vi "Exercício 4.vi"() -> ()   [LabVIEW 2016]
uses:
  bcf247fc-8029-4b24-a8d5-3c8da93c177a.vi
  <vilib>/numeric/Random Number (Range) DBL.vi
  <vilib>/picture/cartesn2.llb/XY Plot Type.ctl
panel:
  in  "dimensions (w,h)":cluster{"width":i16, "height":i16}={"width"=500, "height"=350}
  in  "cartesian grid cosmetics":T1={"line color"=12369084, "text color"=0, "tick length(3)"=3, "crossing axes"=FALSE, "visible grid?"=TRUE}
  in  "cartesian axis attributes":T2={"x minimum"=0.0, "x maximum"=0.0, "x log?"=FALSE, "x precision"=1, "x format"=enum."Scientific", "y minimum"=0.0, "y maximum"=0.0, "y log?"=FALSE, "y precision"=1, "y format"=enum."Decimal"} {"x minimum" format="%0.2f"; "x maximum" format="%0.2f"; "y minimum" format="%0.2f"; "y maximum" format="%0.2f"}
  in  "Slide":dbl(slide) scale=0.0..300.0
  out "Número Aleatório":dbl
  in  "XY plot cosmetics":T4={"plot color"=0, "XY plot type"=enum."connected circles", "baseline"=0.0} {"baseline" format="%0.2f"}
  out "Temperatura vs Tempo":picture
  in  "stop":bool
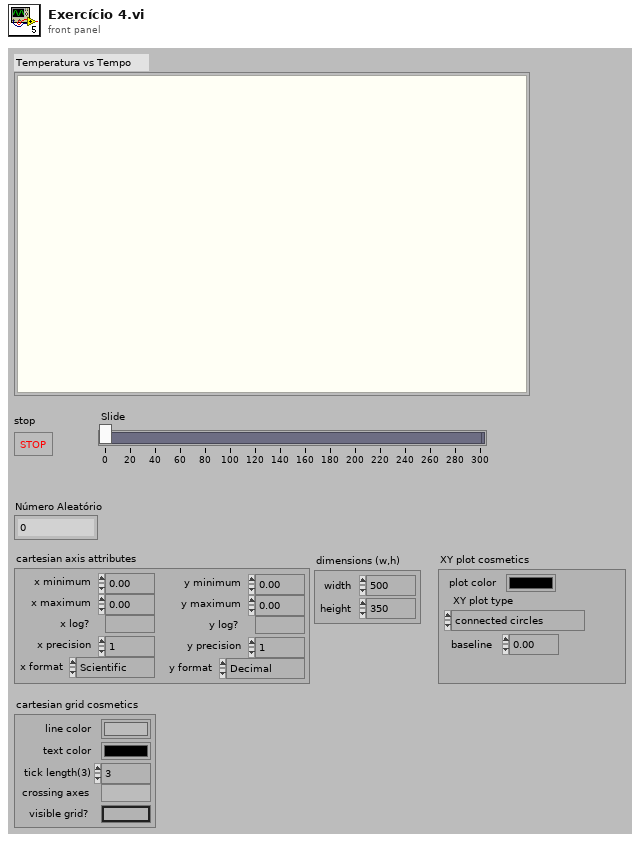
[diagram p1: front panel]
types:
  T1 = cluster{"line color":u32, "text color":u32, "tick length(3)":i16, "crossing axes":bool, "visible grid?":bool}
  T2 = cluster{"x minimum":dbl, "x maximum":dbl, "x log?":bool, "x precision":u8, "x format":enum8{"Decimal", "Scientific", "Engineering", "Binary", "Octal", "Hex"}, "y minimum":dbl, "y maximum":dbl, "y log?":bool, "y precision":u8, "y format":enum8{"Decimal", "Scientific", "Engineering", "Binary", "Octal", "Hex"}}
  T3 = typedef "XY Plot Type.ctl" = enum16{"points", "squares", "circles", "connected points", "connected squares", "connected circles", "comb plot", "sized scatter plot", "sized-colored scatter plot", "min-max lines"}
  T4 = cluster{"plot color":u32, "XY plot type":T3, "baseline":dbl}
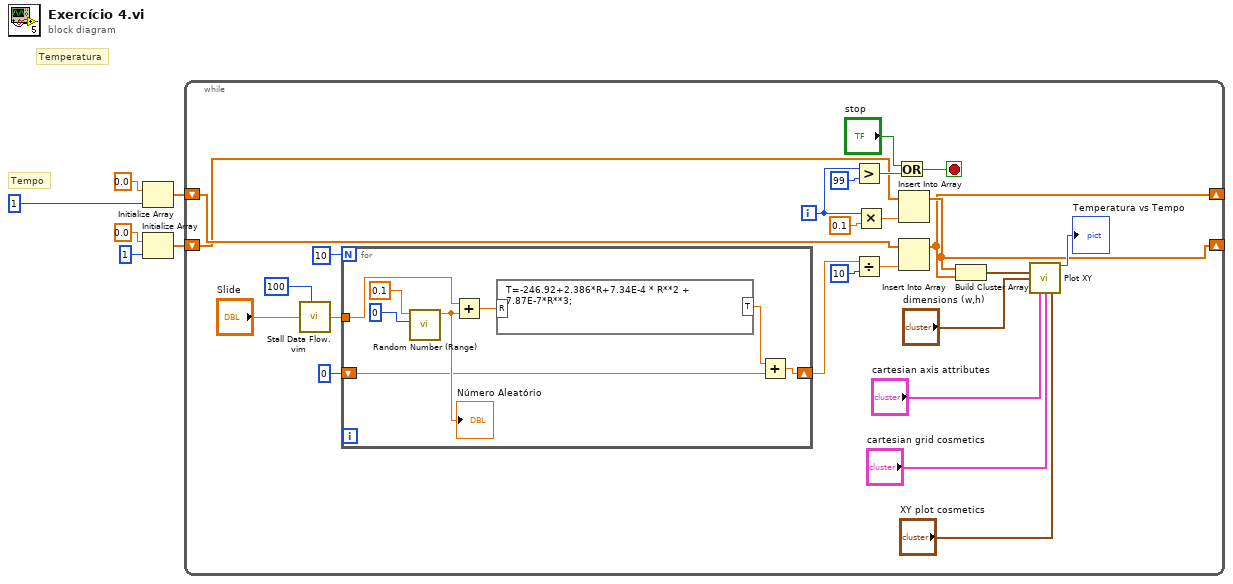
[diagram p0: block diagram]
diagram:
  # "Tempo"
  # "Temperatura"
  n1 = Initialize Array(0.0, 1) -> (w2:dbl[])
  n2 = Initialize Array(0.0, 1) -> (w1:dbl[])
  n3 = while {
    shift-right: [w12] -> _
    shift-left: w2 -> [w19]
    shift-right: [w13] -> _
    shift-left: w1 -> [w17]
    i -> [w20]
    stop <- w22 stop-if-true
    n4 = call "Stall Data Flow.vim"("value in"="Slide", "milliseconds to wait"=100) -> ("value out"=w27:dbl)  [unwired: 1 out]
    n5 = for {
      N: 10 -> [_]
      tunnel: w27 -> [w35]
      shift-right: [w32] -> w30
      shift-left: 0 -> [w33]
      n6 = call-poly <vilib>:"Random Number (Range).vi"("lower bound (0)"=0, "upper bound (100)"=0.1) -> ("number"=w38:dbl)  [unwired: 9 in]
      "Número Aleatório" <- w38
      n7 = Add(x=w35, y=w38) -> (x+y=w39:dbl)
      n8 = formula code="T=-246.92+2.386*R+7.34E-4 * R**2 + 7.87E-7*R**3;"("R"=w39) -> ("T"=w34:dbl)
      n9 = Add(x=w34, y=w33) -> (x+y=w32:dbl)
    }
    n10 = Greater?(x=w20, y=99) -> (0:w24:bool)
    n11 = Divide(x=w30, y=10) -> (x/y=w18:dbl)
    n12 = Multiply(x=w20, y=0.1) -> (x*y=w16:dbl)
    n13 = Or(x="stop", y=w24) -> (x .or. y?=w22:bool)
    n14 = Insert Into Array(array=w17, new element=w16) -> (w13:dbl[])  [unwired: 1 in]
    n15 = Insert Into Array(array=w19, new element=w18) -> (w12:dbl[])  [unwired: 1 in]
    n16 = Build Cluster Array(w13, w12) -> (w15:cluster{dbl, dbl}[])
    n17 = call <vilib>:"Plot XY.vi"("data"=w15, "dimensions (w,h)"="dimensions (w,h)", "cartesian axis attributes"="cartesian axis attributes", "cartesian grid cosmetics"="cartesian grid cosmetics", "XY plot cosmetics"="XY plot cosmetics") -> ("new picture"=→"Temperatura vs Tempo":picture)  [unwired: 10 in]
  }
